vi "Example_guider_Prenom.vi"() -> ()   [LabVIEW 2018]
panel:
  out "array":string[](array[string])
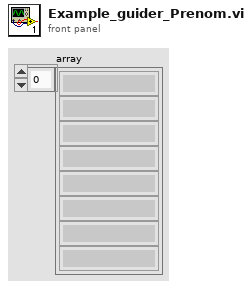
[diagram p1: front panel]
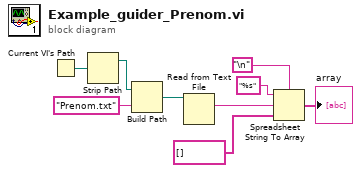
[diagram p0: block diagram]
diagram:
  n1 = Current VI's Path() -> (path=w9:path)
  n2 = Strip Path(path=w9) -> (stripped path=w8:path)  [unwired: 1 out]
  n3 = Build Path(base path=w8, name or relative path="Prenom.txt") -> (appended path=w6:path)
  n4 = Read from Text File(file (use dialog)=w6) -> (text=w4:string)  [unwired: 3 in, 3 out]
  n5 = Spreadsheet String To Array(delimiter (Tab)="\n", format string="%s", spreadsheet string=w4, array type (2D Dbl)=string[] []) -> (array=→"array":string[])
